vi "monitor_wm.vi"() -> ()   [LabVIEW 2009]
panel:
  out "791 Frequency":dbl format="%#_9g"
  in  "791 Channel":i32
  out "Current Channel":i32
  in  "Blue Channel":i32
  out "Waveform Chart 2":dbl(graph)
  in  "Red Channel":i32
  out "Waveform Chart":dbl(graph)
  in  "stop":bool
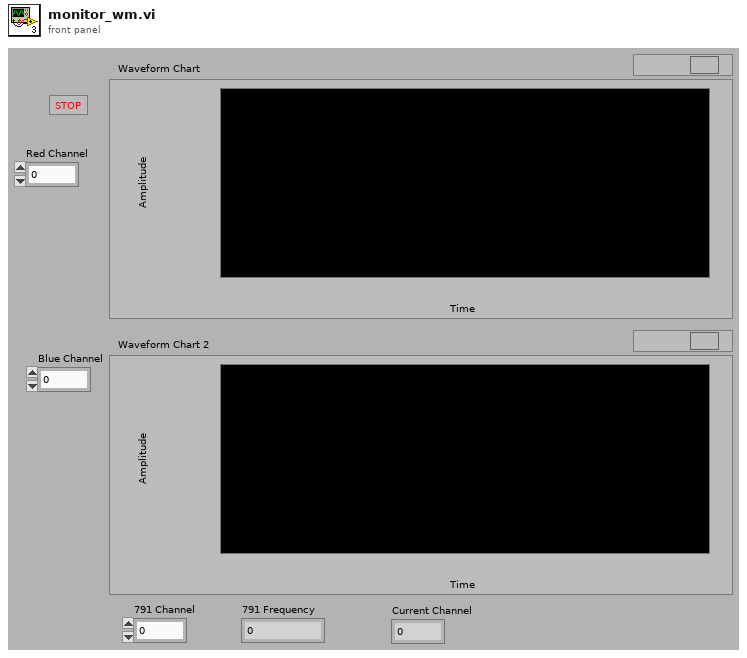
[diagram p1: front panel]
types:
  T1 = enum16{"Read", "Write", "ReadWrite", "BufferedRead", "BufferedReadWrite"}
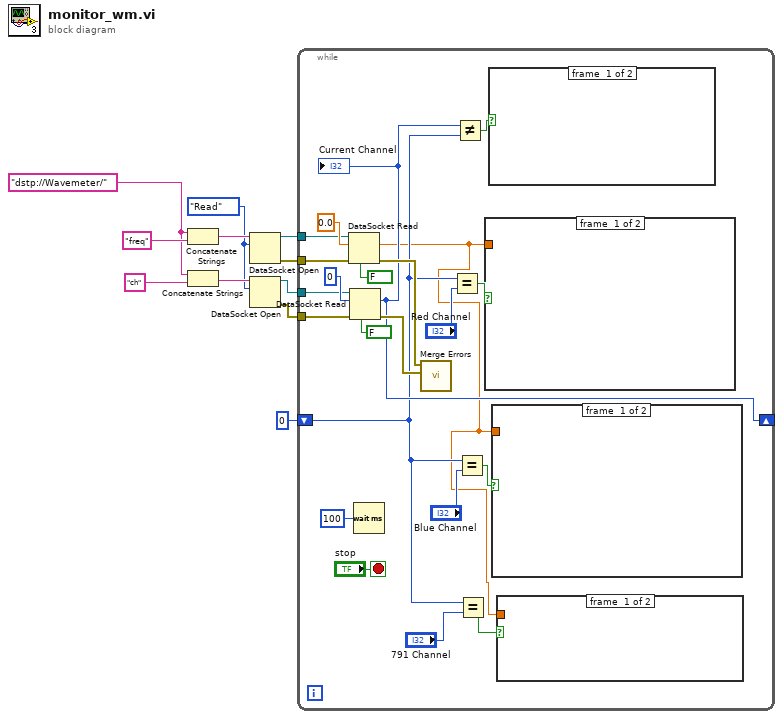
[diagram p0: block diagram]
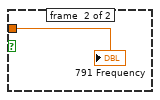
[diagram p2: hidden frame]
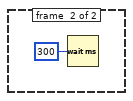
[diagram p3: hidden frame]
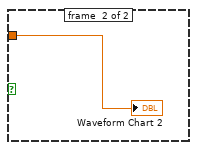
[diagram p4: hidden frame]
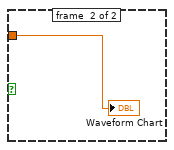
[diagram p5: hidden frame]
diagram:
  w6 = T1."Read" ("mode")
  w7 = "dstp://Wavemeter/" ("string")
  n1 = Concatenate Strings(w7, "freq" ("string")) -> (w9:string)
  n2 = Concatenate Strings(w7, "ch" ("string")) -> (w8:string)
  n3 = DataSocket Open(10:w6, 11:w9) -> (0:w2:errorcluster, 3:w5:refnum<k13>)  [unwired: 2 in]
  n4 = DataSocket Open(10:w6, 11:w8) -> (0:w3:errorcluster, 3:w4:refnum<k13>)  [unwired: 2 in]
  n5 = while {
    tunnel: w5 -> [w26]
    tunnel: w4 -> [w25]
    tunnel: w3 -> [w24]
    tunnel: w2 -> [w23]
    shift-right: [w17] -> _
    shift-left: 0 ("Cur Ch") -> [w15]
    stop <- "stop" stop-if-true
    n6 = DataSocket Read(6:FALSE ("wait for updated value (T)"), 8:w23, 10:0.0 ("Frequency"), 11:w26) -> (0:w31:errorcluster, 2:w13:dbl)  [unwired: 1 in, 5 out]
    n7 = DataSocket Read(6:FALSE ("wait for updated value (T)"), 8:w24, 10:0 ("Cur Ch"), 11:w25) -> (0:w30:errorcluster, 2:w17:i32)  [unwired: 1 in, 5 out]
    "Current Channel" <- w17
    n8 = Wait (ms)(milliseconds to wait=u32 100) -> ()  [unwired: 1 out]
    n9 = call <vilib>:"Merge Errors.vi"("error in 2 (no error)"=w30, "error in 1 (no error)"=w31) -> ()  [unwired: 5 in, 1 out]
    n10 = Equal?(x=w15, y="Red Channel") -> (x = y?=w22:bool)
    n11 = Not Equal?(x=w17, y=w15) -> (x != y?=w16:bool)
    n12 = Equal?(x=w15, y="Blue Channel") -> (x = y?=w18:bool)
    n13 = Equal?(x=w15, y="791 Channel") -> (x = y?=w12:bool)
    n14 = case shown="True" w22 {
      tunnel: w13 -> [_ w37]
      frame #0 {
      }
      frame #1 {
        "Waveform Chart" <- w37
      }
    }
    n15 = case shown="True" w16 {
      frame #0 {
      }
      frame #1 {
        n16 = Wait (ms)(milliseconds to wait=u32 300) -> ()  [unwired: 1 out]
      }
    }
    n17 = case shown="True" w18 {
      tunnel: w13 -> [_ w36]
      frame #0 {
      }
      frame #1 {
        "Waveform Chart 2" <- w36
      }
    }
    n18 = case shown="True" w12 {
      tunnel: w13 -> [_ w34]
      frame #0 {
      }
      frame #1 {
        "791 Frequency" <- w34
      }
    }
  }
